vi "De-NaN Values.vi"(10 "Last Valid":dbl, 11 "Input":dbl) -> (3 "De-NaN":dbl)   [LabVIEW 2016]
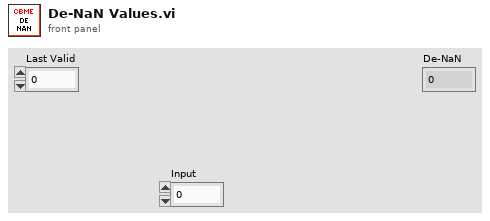
[diagram p1: front panel]
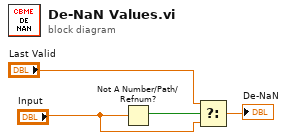
[diagram p0: block diagram]
diagram:
  n1 = Not A Number/Path/Refnum?(number/path/refnum="Input") -> (NaN/Path/Refnum?=w1:bool)
  n2 = Select(t="Last Valid", s=w1, f="Input") -> (s? t:f=→"De-NaN":dbl)
